vi "Discrete FP Transfer Function to FXP.vi"(8 "error in (no error)":errorcluster, 11 "FP Transfer Function Model":T1 {"Denominator" format="%#_9g"; "Numerator" format="%#_9g"}) -> (0 "error out":errorcluster, 3 "FXP Transfer Function Model":T2)   [LabVIEW 2020, in "NI_FpgaMspHost.lvlib"]
doc: "Converts a transfer function system model from floating-point to fixed-point representation. Obtain this model by entering values into the <B>FP Transfer Function Model</B> control or by using the VIs included with the LabVIEW Control Design & Simulation Module.You then can implement this model on an FPGA by using the Discrete Transfer Function Direct VI."
uses:
  <vilib>/rvi/Analysis/host/Public/NI_FpgaMspHost.lvlib
  <vilib>/rvi/Analysis/control/linear/templates/niFPGA FXP Transfer Function Model.ctl
  <vilib>/Simulation/Shared/_Datatypes/SIM SISO Transfer Function.ctl
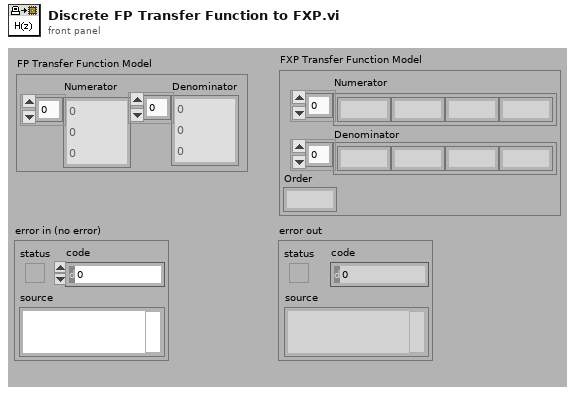
[diagram p1: front panel]
types:
  T1 = typedef "SIM SISO Transfer Function.ctl" = cluster{"Numerator":dbl[], "Denominator":dbl[]}
  T2 = typedef "niFPGA FXP Transfer Function Model.ctl" = cluster{"Numerator":fxp<+/-,32,12>[], "Denominator":fxp<+/-,32,12>[], "Order":u8}
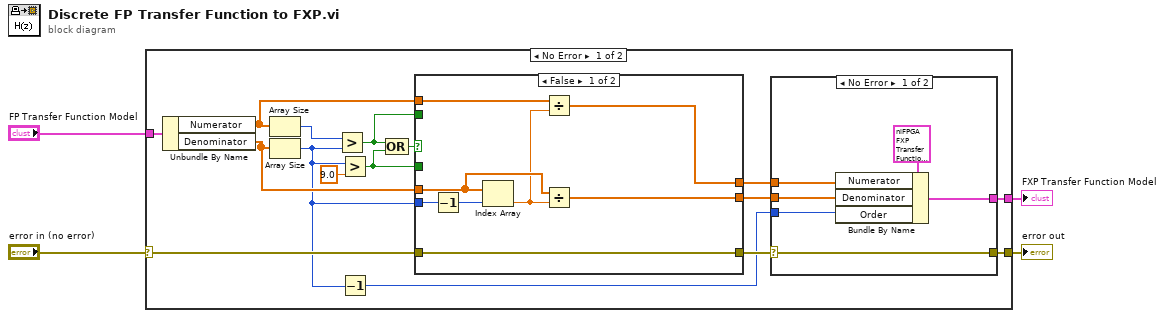
[diagram p0: block diagram]
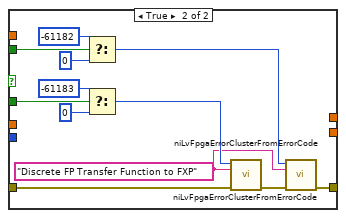
[diagram p3: hidden frame]
diagram:
  n1 = case shown="No Error" "error in (no error)" {
    selector: "error in (no error)" -> [w18 w48]
    tunnel: [w11 w48] -> w3
    tunnel: "FP Transfer Function Model" -> [w20 _]
    tunnel: [w9 _] -> w1
    frame No Error {
      n2 = Unbundle By Name(w20) -> ("Numerator"=w8:dbl[], "Denominator"=w13:dbl[])
      n3 = Array Size(array=w8) -> (size(s)=w19:i32)
      n4 = Array Size(array=w13) -> (size(s)=w6:i32)
      n5 = Greater?(x=w19, y=w6) -> (0:w15:bool)
      n6 = Greater?(x=w6, y=9.0) -> (0:w14:bool)
      n7 = Decrement(x=w6) -> (x-1=w5:i32)
      n8 = Compound Arithmetic op=OR(w15, w14) -> (w16:bool)
      n9 = case shown="False" w16 {
        tunnel: [w35 w36] -> w12
        tunnel: w18 -> [w35 w47]
        tunnel: w15 -> [_ w46]
        tunnel: w14 -> [_ w40]
        tunnel: w13 -> [w33 _]
        tunnel: w6 -> [w34 _]
        tunnel: [w32 _] -> w10
        tunnel: w8 -> [w30 _]
        tunnel: [w28 _] -> w7
        frame False {
          n10 = Decrement(x=w34) -> (x-1=w31:i32)
          n11 = Index Array(array=w33, index=w31) -> (element=w29:dbl)
          n12 = Divide(x=w30, y=w29) -> (x/y=w28:dbl[])
          n13 = Divide(x=w33, y=w29) -> (x/y=w32:dbl[])
        }
        frame True {
          w38 = "Discrete FP Transfer Function to FXP" ("L10N_Function Name")
          n14 = Select(t=-61182 ("error code"), s=w46, f=0) -> (s? t:f=w37:i32)
          n15 = Select(t=-61183 ("error code"), s=w40, f=0) -> (s? t:f=w39:i32)
          n16 = call <vilib>:"niLvFpgaErrorClusterFromErrorCode.vi"("error code"=w39, "function name"=w38, "error in"=w47) -> ("error out"=w43:errorcluster)  [unwired: 4 in, 8 out]
          n17 = call <vilib>:"niLvFpgaErrorClusterFromErrorCode.vi"("error code"=w37, "function name"=w38, "error in"=w43) -> ("error out"=w36:errorcluster)  [unwired: 4 in, 8 out]
        }
      }
      n18 = case shown="No Error" w12 {
        selector: w12 -> [w26 w27]
        tunnel: [w26 w27] -> w11
        tunnel: w10 -> [w24 _]
        tunnel: w7 -> [w25 _]
        tunnel: [w23 _] -> w9
        tunnel: w5 -> [w22 _]
        frame No Error {
          n19 = Bundle By Name(cluster=T2 {"Numerator"=[0.0, 0.0, 0.0, 0.0, 0.0, 0.0, 0.0, 0.0, 0.0], "Denominator"=[0.0, 0.0, 0.0, 0.0, 0.0, 0.0, 0.0, 0.0, 0.0], "Order"=0} ("FXP Transfer Function Model"), "Numerator"=w25, "Denominator"=w24, "Order"=w22) -> (w23:T2)
        }
        frame Error {
        }
      }
    }
    frame Error {
    }
  }
  "FXP Transfer Function Model" <- w1
  "error out" <- w3
